vi "update mode in ui.vi"(8 "error in (no error)":errorcluster caption="에러 입력(에러 없음)", 10 "mode":T1, 11 "DW7914 입력":refnum<class "DW7914.lvclass">) -> (0 "error out":errorcluster caption="에러 출력", 3 "DW7914 출력":refnum<class "DW7914.lvclass">)   [LabVIEW 2020, in "DW7914.lvclass"]
uses:
  DW7914.lvclass
  Haptic IC/Controls/(Ctrl)Mode.ctl
  Haptic IC/Haptic IC.lvclass/Haptic IC.ctl
  Haptic IC/Accessors/Read mode ref.vi
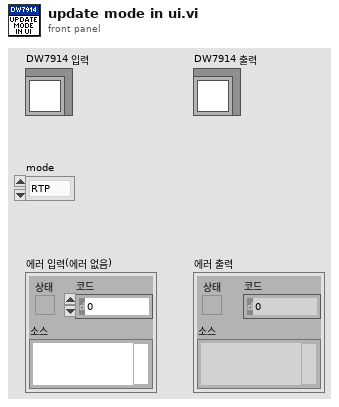
[diagram p1: front panel]
types:
  T1 = typedef "(Ctrl)Mode.ctl" = enum16{"RTP", "Memory"}
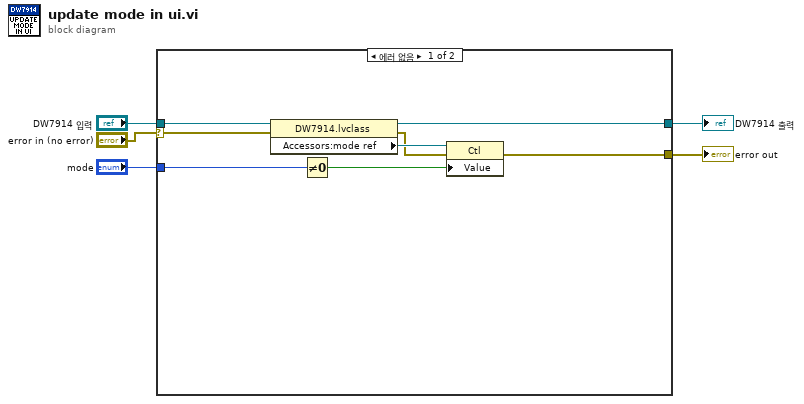
[diagram p0: block diagram]
diagram:
  n1 = case shown="에러 없음" "error in (no error)" {
    selector: "error in (no error)" -> [w13 w14]
    tunnel: "DW7914 입력" -> [w12 w15]
    tunnel: [w8 w14] -> w5
    tunnel: [w11 w15] -> w1
    tunnel: "mode" -> [w7 _]
    frame No Error {
      n2 = property class="DW7914.lvclass"(reference=w12, error in=w13) -> (reference out=w11:refnum<class "DW7914.lvclass">, error out=w9:errorcluster, "Accessors:mode ref"=w10:refnum<vi>)
      n3 = Not Equal To 0?(x=w7) -> (x != 0?=w6:bool)
      n4 = property class="Ctl"(reference=w10, error in=w9, "Value"=w6) -> (error out=w8:errorcluster)  [unwired: 1 out]
    }
    frame Error {
    }
  }
  "error out" <- w5
  "DW7914 출력" <- w1
